vi "read_buffer.vi"(11 "buffer":string) -> (0 "ACS712-30A value":dbl, 1 "potentiometer value":dbl, 2 "BMP180 value":dbl, 3 "DS18B20 value":dbl, 4 "Voltage in range?":bool, 5 "Pressure in range?":bool, 6 "Amperage in range?":bool, 7 "Temperature in range?":bool)   [LabVIEW 2016]
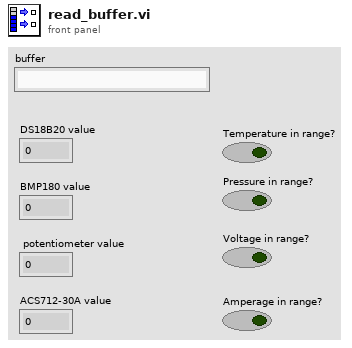
[diagram p1: front panel]
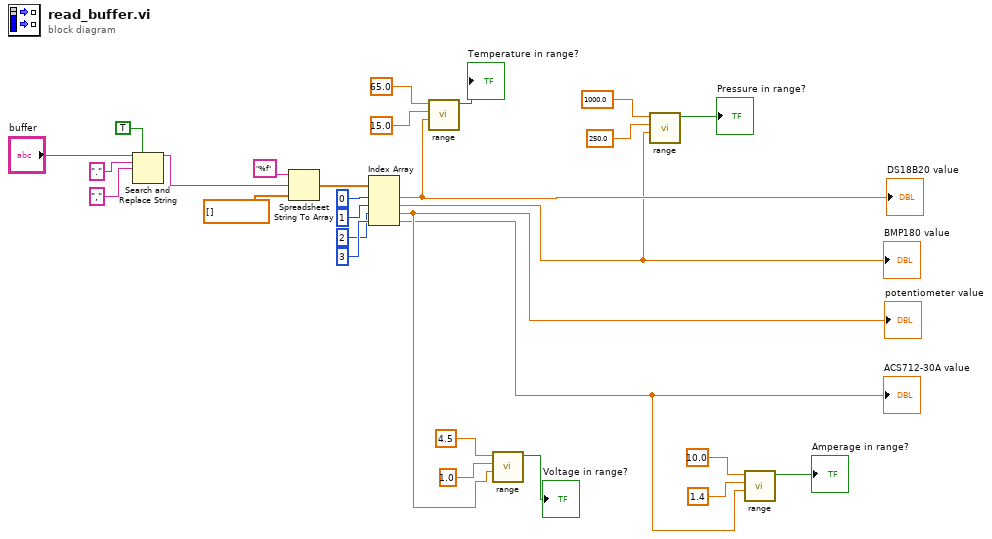
[diagram p0: block diagram]
diagram:
  n1 = Search and Replace String(replace all?=TRUE ("replace all? (F)"), input string="buffer", search string="." ("replace string (\"\")"), replace string="," ("replace string (\"\")")) -> (result string=w19:string)  [unwired: 4 in, 3 out]
  n2 = Spreadsheet String To Array(format string="%f", spreadsheet string=w19, array type (2D Dbl)=dbl[] []) -> (array=w23:dbl[])  [unwired: 1 in]
  n3 = Index Array(array=w23, index #1=0 ("index"), index #2=1 ("index"), index #3=2 ("index"), index #4=3 ("index")) -> (element #1=w13:dbl, element #2=w9:dbl, element #3=w5:dbl, element #4=w1:dbl)
  "ACS712-30A value" <- w1
  "potentiometer value" <- w5
  "BMP180 value" <- w9
  "DS18B20 value" <- w13
  n4 = call "range.vi"("Value"=w13, "lower limit"=15.0, "upper limit"=65.0) -> ("In range?"=→"Temperature in range?":bool)  [unwired: 8 in]
  n5 = call "range.vi"("Value"=w5, "lower limit"=1.0, "upper limit"=4.5) -> ("In range?"=→"Voltage in range?":bool)  [unwired: 8 in]
  n6 = call "range.vi"("Value"=w9, "lower limit"=250.0, "upper limit"=1000.0) -> ("In range?"=→"Pressure in range?":bool)  [unwired: 8 in]
  n7 = call "range.vi"("Value"=w1, "lower limit"=1.4, "upper limit"=10.0) -> ("In range?"=→"Amperage in range?":bool)  [unwired: 8 in]
